vi "configure scope.vi"(8 "error in":errorcluster, 10 "Init cluster":T1, 11 "VISA resource name I":refnum<visa-resource-name>) -> (0 "error out":errorcluster, 2 "ready":bool, 3 "VISA resource name O":refnum<visa-resource-name>)   [LabVIEW 2026]
uses:
  <instrlib>/Agilent 2000 3000 X-Series/Agilent 2000 3000 X-Series.lvlib
  <instrlib>/Agilent 2000 3000 X-Series/Public/Configure/Configure Timebase (Basic).vi
  <instrlib>/Agilent 2000 3000 X-Series/Public/Configure/Trigger/Configure Trigger (Edge).vi
  controls/init cluster.ctl
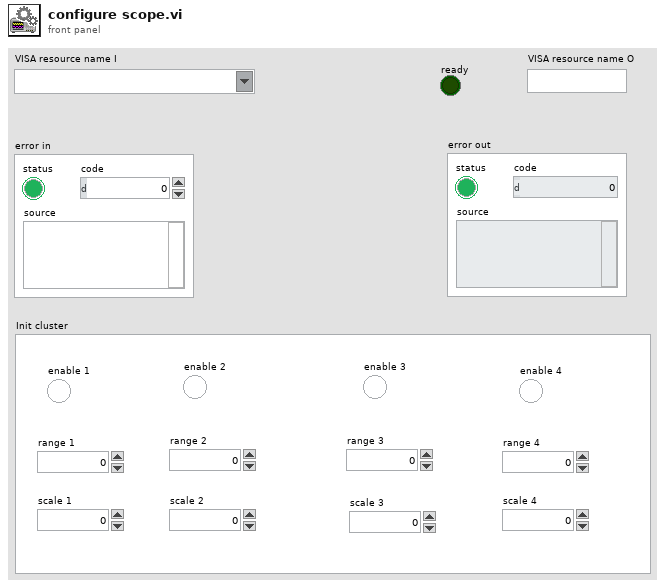
[diagram p1: front panel]
types:
  T1 = typedef "init cluster.ctl" = cluster{"enable 1":bool, "enable 2":bool, "enable 3":bool, "enable 4":bool, "range 1":dbl, "range 2":dbl, "range 3":dbl, "range 4":dbl, "scale 1":dbl, "scale 2":dbl, "scale 3":dbl, "scale 4":dbl}
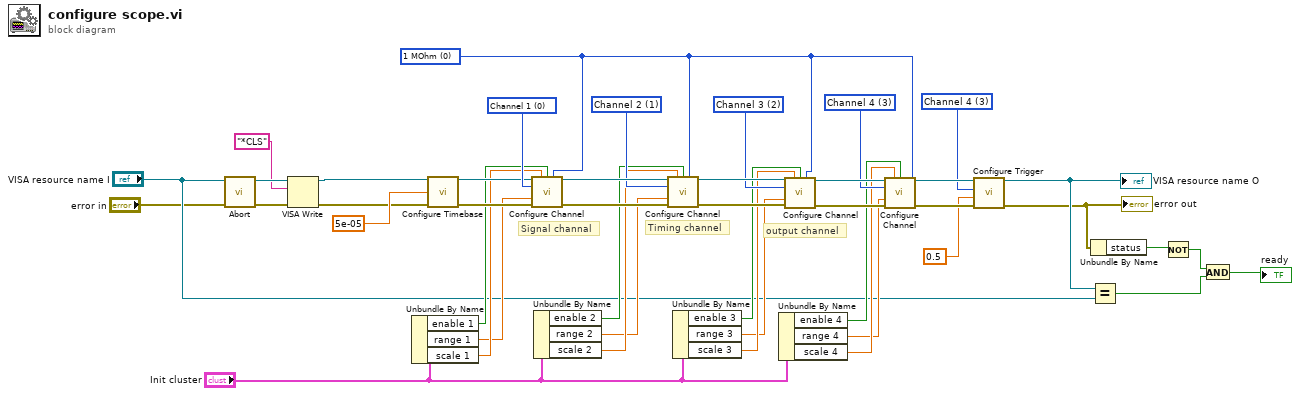
[diagram p0: block diagram]
diagram:
  w24 = 3 items=["Channel 1"=0, "Channel 2"=1, "Channel 3"=2, "Channel 4"=3, "D0"=13, "D1"=14, "D2"=15, "D3"=16, "D4"=17, "D5"=18, "D6"=19, "D7"=20, "D8"=21, "D9"=22, "D10"=23, "D11"=24, "D12"=25, "D13"=26, "D14"=27, "D15"=28, "External"=29, "Power Line"=30, "Waveform Generator"=31, "Waveform Generator1"=32, "Waveform Modulation"=33, "Waveform Generator2"=34] ("Trigger Source (0: Channel 1)")
  w29 = 0 items=["1 MOhm", "50 Ohm"] ("Impedance (0: 1 MOhm)")
  w34 = 3 items=["Channel 1", "Channel 2", "Channel 3", "Channel 4"] ("Channel Name (0: Channel 1)")
  w37 = 2 items=["Channel 1", "Channel 2", "Channel 3", "Channel 4"] ("Channel Name (0: Channel 1)")
  w40 = 1 items=["Channel 1", "Channel 2", "Channel 3", "Channel 4"] ("Channel Name (0: Channel 1)")
  w43 = 0 items=["Channel 1", "Channel 2", "Channel 3", "Channel 4"] ("Channel Name (0: Channel 1)")
  # "output channel"
  # "Timing channel"
  # "Signal channal"
  n1 = call <instrlib>:"Abort.vi"("error in (no error)"="error in", "VISA resource name"="VISA resource name I") -> ("error out"=w4:errorcluster, "VISA resource name out"=w5:refnum<visa-resource-name>)  [unwired: 8 in]
  n2 = VISA Write(VISA resource name=w5, write buffer="*CLS", error in (no error)=w4) -> (VISA resource name out=w2:refnum<visa-resource-name>, error out=w3:errorcluster)  [unwired: 1 out]
  n3 = Unbundle By Name("Init cluster") -> ("enable 1"=w19:bool, "range 1"=w17:dbl, "scale 1"=w18:dbl)
  n4 = call-poly <instrlib>:"Configure Timebase.vi"("VISA resource name"=w2, "Scale (50 s/div)"=5e-05, "error in (no error)"=w3) -> ("VISA resource name out"=w22:refnum<visa-resource-name>, "error out"=w23:errorcluster)  [unwired: 11 in]
  n5 = call <instrlib>:"Configure Channel.vi"("VISA resource name"=w22, "Vertical Scale (5.0 V)"=w18, "Enable Channel (T: Enable)"=w19, "Impedance (0: 1 MOhm)"=w29, "Channel Name (0: Channel 1)"=w43, "Vertical Range (40.0 V)"=w17, "error in (no error)"=w23) -> ("VISA resource name out"=w42:refnum<visa-resource-name>, "error out"=w41:errorcluster)  [unwired: 7 in]
  n6 = Unbundle By Name("Init cluster") -> ("enable 2"=w16:bool, "range 2"=w14:dbl, "scale 2"=w15:dbl)
  n7 = call <instrlib>:"Configure Channel.vi"("VISA resource name"=w42, "Vertical Scale (5.0 V)"=w15, "Enable Channel (T: Enable)"=w16, "Impedance (0: 1 MOhm)"=w29, "Channel Name (0: Channel 1)"=w40, "Vertical Range (40.0 V)"=w14, "error in (no error)"=w41) -> ("VISA resource name out"=w39:refnum<visa-resource-name>, "error out"=w38:errorcluster)  [unwired: 7 in]
  n8 = Unbundle By Name("Init cluster") -> ("enable 3"=w13:bool, "range 3"=w11:dbl, "scale 3"=w12:dbl)
  n9 = Unbundle By Name("Init cluster") -> ("enable 4"=w10:bool, "range 4"=w8:dbl, "scale 4"=w9:dbl)
  n10 = call <instrlib>:"Configure Channel.vi"("VISA resource name"=w39, "Vertical Scale (5.0 V)"=w12, "Enable Channel (T: Enable)"=w13, "Impedance (0: 1 MOhm)"=w29, "Channel Name (0: Channel 1)"=w37, "Vertical Range (40.0 V)"=w11, "error in (no error)"=w38) -> ("VISA resource name out"=w36:refnum<visa-resource-name>, "error out"=w35:errorcluster)  [unwired: 7 in]
  n11 = call <instrlib>:"Configure Channel.vi"("VISA resource name"=w36, "Vertical Scale (5.0 V)"=w9, "Enable Channel (T: Enable)"=w10, "Impedance (0: 1 MOhm)"=w29, "Channel Name (0: Channel 1)"=w34, "Vertical Range (40.0 V)"=w8, "error in (no error)"=w35) -> ("VISA resource name out"=w27:refnum<visa-resource-name>, "error out"=w28:errorcluster)  [unwired: 7 in]
  n12 = call-poly <instrlib>:"Configure Trigger.vi"("error in (no error)"=w28, "Trigger Level (0 V)"=0.5, "Trigger Source (0: Channel 1)"=w24, "VISA resource name"=w27) -> ("error out"=w25:errorcluster, "VISA resource name out"=w26:refnum<visa-resource-name>)  [unwired: 6 in]
  "VISA resource name O" <- w26
  "error out" <- w25
  n13 = Equal?(x=w26, y="VISA resource name I") -> (x = y?=w31:bool)
  n14 = Unbundle By Name(w25) -> ("status"=w33:bool)
  n15 = Not(x=w33) -> (.not. x?=w32:bool)
  n16 = And(x=w32, y=w31) -> (x .and. y?=→"ready":bool)
